vi "Sync (SubVI).vi"(11 "sampled\n   array":cdb[](array[numeric])) -> (3 "after_sync":cdb[](array[numeric]))   [LabVIEW 2015]
uses:
  <vilib>/Analysis/2dsp.llb/1D Cross Correlation (CDB).vi
  <vilib>/imath/engines/lvmath2/RunTimeEngine/ErrorHandling/NIMS_Finalize Error.vi
  <vilib>/Analysis/NI_AALPro.lvlib
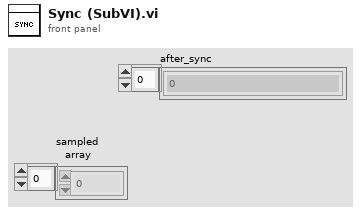
[diagram p1: front panel]
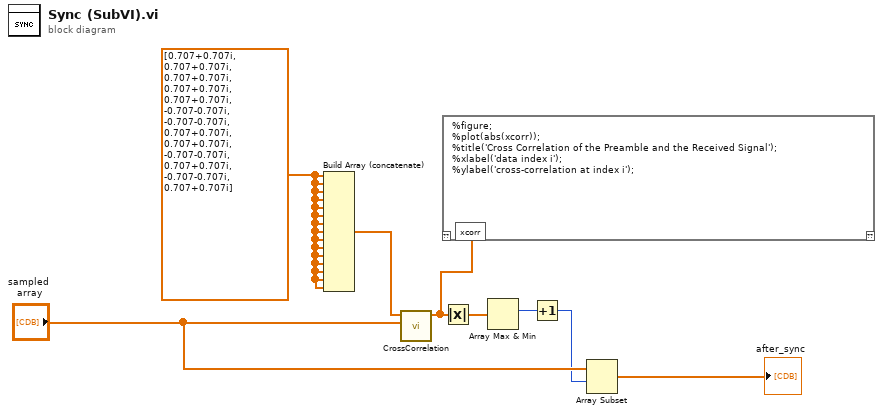
[diagram p0: block diagram]
diagram:
  w3 = cdb[] [0.707+0.707i, 0.707+0.707i, 0.707+0.707i, 0.707+0.707i, 0.707+0.707i, -0.707-0.707i, -0.707-0.707i, 0.707+0.707i, 0.707+0.707i, -0.707-0.707i, 0.707+0.707i, -0.707-0.707i, 0.707+0.707i] ("array 2")
  n1 = Build Array (concatenate)(w3, w3, w3, w3, w3, w3, w3, w3, w3, w3, w3, w3, w3, w3, w3) -> (w2:cdb[])
  n2 = call-poly <vilib>:"CrossCorrelation.vi"("Y"="sampled\n   array", "X"=w2) -> ("Rxy"=w4:cdb[])  [unwired: 8 in, 1 out]
  n3 = mathscript code="%figure;\n%plot(abs(xcorr));\n%title('Cross Correlation of the Preamble and the Received Signal');\n%xlabel('data index i');\n%ylabel('cross-correlation at index i');"("xcorr"=w4) -> ()  [unwired: 1 in, 1 out]
  n4 = Absolute Value(x=w4) -> (abs(x)=w7:dbl[])
  n5 = Array Max & Min(array=w7) -> (max index (indices)=w6:i32)  [unwired: 3 out]
  n6 = Increment(x=w6) -> (x+1=w1:i32)
  n7 = Array Subset(array="sampled\n   array", index=w1) -> (→"after_sync":cdb[])  [unwired: 1 in]
